vi "DBeditSendDataToServer.vi"(8 "error in (no error)":errorcluster, 9 "data":variant, 10 "Query_type":T1, 11 "Gviewer in":refnum<class "DB-editor.lvclass">) -> (0 "error out":errorcluster, 3 "Gviewer out":refnum<class "DB-editor.lvclass">)   [LabVIEW 2020, in "Sgraph_lib_V1.lvlib" / "DB-editor.lvclass"]
doc: "Andre Koelewijn, 5 jan 2021\n\nSend Request to Gserver Queue"
uses:
  DB-editor.lvclass
  Gserver/controls/Typedef_QueryType.ctl
  Gserver/controls/Typedef_Gviewer-Query.ctl
  DB-editor.lvclass/DB-editor.ctl
  Gserver/Gserver.lvclass
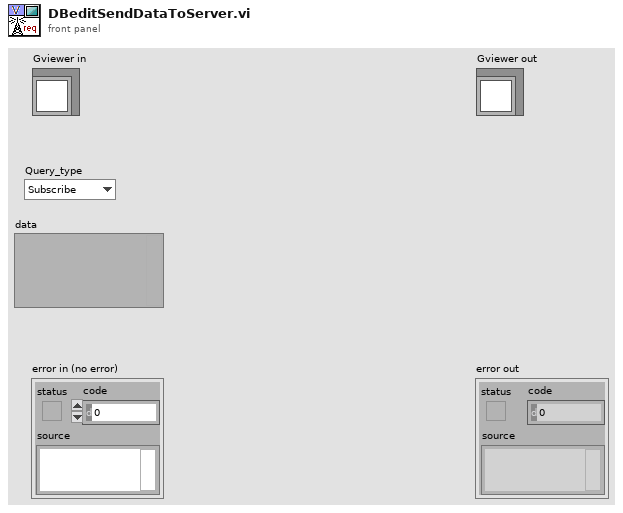
[diagram p1: front panel]
types:
  T1 = typedef "Sgraph_lib_V1.lvlib/Gserver.lvclass/Typedef_QueryType.ctl" = enum16{"Subscribe", "DataRequest", "RequestAllTags", "RequestIniPath", "FAMMstarted", "SetClientOptions", "GviewerUpdate", "OpenNewGraph", "CloseClient", "CloseAllClients", "Close Gserver", "OpenMemoryMap", "MeMapDataRequest", "MeMapDataResponse", "OpenDBeditor", "CheckDBeditorRunning", "StoppedDBeditor", "SaveDB_TAGpropRecord", "ConfirmDB_TAGpropSave", "GetXconstraints"}
  T2 = typedef "Sgraph_lib_V1.lvlib/Gserver.lvclass/Typedef_Gviewer-Query.ctl" = cluster{"Query_type":T1, "data":variant, "Source":string, "Time Stamp":timestamp}
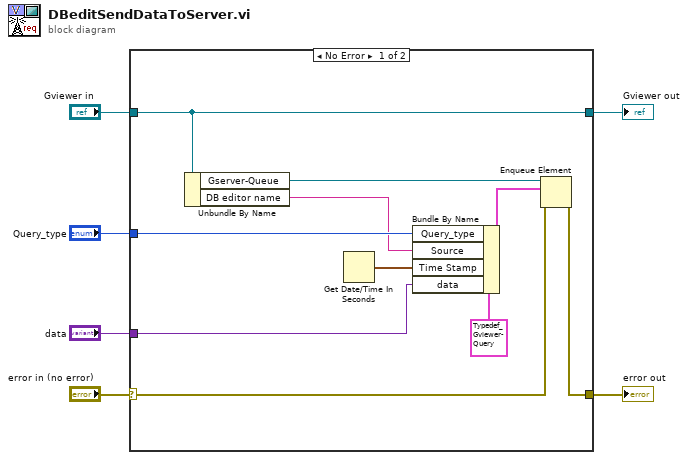
[diagram p0: block diagram]
diagram:
  n1 = case shown="No Error" "error in (no error)" {
    selector: "error in (no error)" -> [w11 w18]
    tunnel: [w10 w18] -> w5
    tunnel: [w12 w17] -> w3
    tunnel: "Gviewer in" -> [w12 w17]
    tunnel: "Query_type" -> [w9 _]
    tunnel: "data" -> [w8 _]
    frame No Error {
      n2 = Unbundle By Name(w12) -> ("Gserver-Queue"=w16:refnum<queue>, "DB editor name"=w7:string)
      n3 = Get Date/Time In Seconds() -> (seconds since 1Jan1904=w14:timestamp)
      n4 = Bundle By Name(cluster=T2 {"Query_type"=enum."Subscribe", "data"=variant, "Source"="", "Time Stamp"=timestamp(0 s since 1904-01-01)} ("element"), "Query_type"=w9, "Source"=w7, "Time Stamp"=w14, "data"=w8) -> (w15:T2)
      n5 = Enqueue Element(queue=w16, element=w15, error in (no error)=w11) -> (error out=w10:errorcluster)  [unwired: 1 in, 2 out]
    }
    frame Error {
    }
  }
  "error out" <- w5
  "Gviewer out" <- w3
